vi "KSF.vi"(0 "System no.":i32=1 min=1 max=4 step=1, 1 "Name":string, 5 "error in":errorcluster) -> (14 "Controller error":bool, 19 "error out":errorcluster)   [LabVIEW 2020]
doc: "Defines a coordinate system based on the current position of the hexapod platform and queries ERR?. \nIf there is already a coordinate system with the same name, KSF will replace it if it is not used. Activating a KSF type coordinate system (KEN.vi) does not cause any motion, and POS?.vi will report position (0, 0, 0 ,0 ,0 ,0). If the hexapod is moving, the command cannot be applied.All pivot point coordinates (SPI.vi) will remain. SPI.vi is allowed when a KSF type coordinate system is active. For new or replaced KSF type coordinate systems, the parent coordinate system will be set to \"ZERO\". When replacing a coordinate system of this type, the chain relations will be changed and the parent will be set to \"ZERO\". Coordinate systems that are currently in use cannot be changed. Coordinate system settings are volatile but can be saved as power-on default with WPA.vi using the password \"SKS\". This command requires command level 0 or 1. Controller error is TRUE if selected system reports error code not equal to 0.\n\nC-887, F-206, M-8X0: Only for GCS syntax version = GCS 2.0 or higher (Check with CSV?.vi. If CSV?.vi is not supported, syntax version is GCS 1.0)."
panel:
  # "Defines a coordinate system based on the current position\nof the Hexapod platform and queries ERR?."
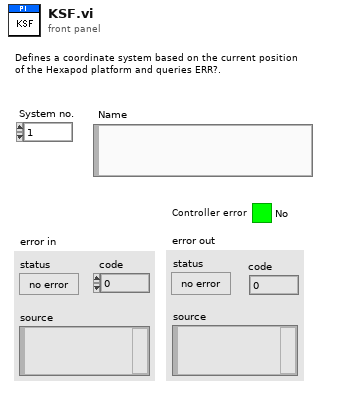
[diagram p1: front panel]
types:
  T1 = enum16{"Disable error check", "Force error check", "Use global settings"}
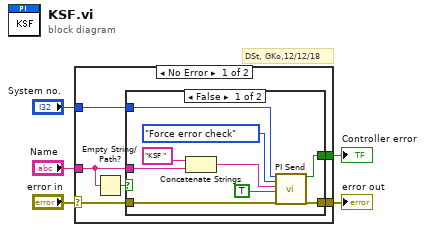
[diagram p0: block diagram]
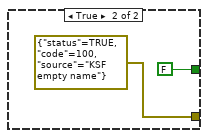
[diagram p2: hidden frame]
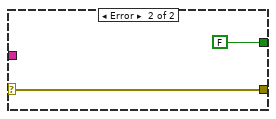
[diagram p3: hidden frame]
diagram:
  # "DSt, GKo,12/12/18"
  n1 = case shown="No Error" "error in" {
    selector: "error in" -> [w6 w23]
    tunnel: [w11 w23] -> w1
    tunnel: [w10 FALSE ("Controller error")] -> w2
    tunnel: "System no." -> [w9 _]
    tunnel: "Name" -> [w7 _]
    frame No Error {
      n2 = Empty String/Path?(string/path=w7) -> (empty?=w8:bool)
      n3 = case shown="False" w8 {
        tunnel: w6 -> [w20 _]
        tunnel: [w14 errorcluster {"status"=TRUE, "code"=100, "source"="KSF empty name"} ("error out")] -> w11
        tunnel: [w15 FALSE ("Controller error")] -> w10
        tunnel: w9 -> [w17 _]
        tunnel: w7 -> [w16 _]
        frame False {
          n4 = Concatenate Strings("KSF ", w16) -> (w18:string)
          n5 = call "PI Send.vi"("System no."=w17, "Error check settings"=T1."Force error check", "String to send"=w18, "Attach termination char.?"=TRUE ("Attach Linefeed?"), "error in"=w20) -> ("Controller error"=w15:bool, "error out"=w14:errorcluster)  [unwired: 1 in, 12 out]
        }
        frame True {
        }
      }
    }
    frame Error {
    }
  }
  "error out" <- w1
  "Controller error" <- w2
